vi "WLAN - Test - UTIL - GetTimeSinceLastCall.vi"(8 "error in (no error)":errorcluster) -> (0 "error out":errorcluster, 4 "Time Since Last Call (s)":dbl)   [LabVIEW 2011]
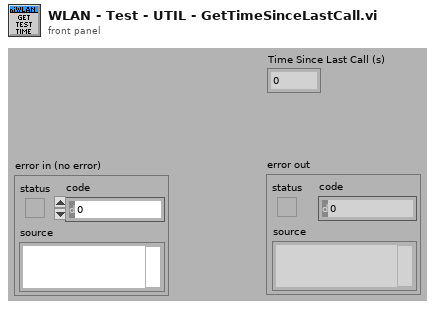
[diagram p1: front panel]
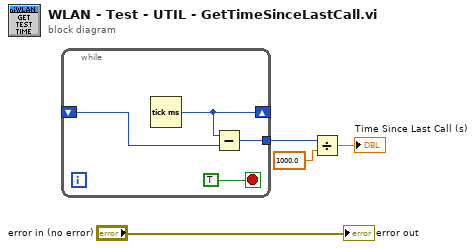
[diagram p0: block diagram]
diagram:
  n1 = while {
    shift-right: [w8] -> _
    shift-left: _ -> [w7]
    tunnel: [w5] -> w1
    stop <- TRUE stop-if-true
    n2 = Tick Count (ms)() -> (millisecond timer value=w8:u32)
    n3 = Subtract(x=w8, y=w7) -> (x-y=w5:u32)
  }
  n4 = Divide(x=w1, y=1000.0) -> (x/y=→"Time Since Last Call (s)":dbl)
  "error out" <- "error in (no error)"
